vi "local FIFO 5 ch 8or12kHz resonance scanner (FPGA) fixed pix clock.vi"() -> ()   [LabVIEW 2012]
uses:
  <vilib>/eio/EIONode/EIONode.xnode
  <vilib>/rvi/eio/common/nirviEmuTemplateMethod_errors.vi
  <vilib>/rvi/DataTransferAndStorage/Container/XNode/niFpgaContainer.xnode
  <vilib>/platform/TimedLoop/XDataNode/XDataNode.xnode
  <vilib>/Platform/TimedLoop/XDataNode/nitl_modes.ctl
  <vilib>/Platform/TimedLoop/XDataNode/XDNodeRunTimeDep.lvlib
  <vilib>/Platform/TimedLoop/XDataNode/wakeup.ctl
  <vilib>/Platform/TimedLoop/XDataNode/timing_clust.ctl
  <vilib>/rvi/interface/RandomDataEmulation/nirviRandomDataFpgaReadWriteTemplate.vi
  <vilib>/rvi/FIFO/Fifo_Resource/nirvififoEmulationRead.vi
  <vilib>/rvi/FIFO/Fifo_Resource/nirvififoEmulationWrite.vi
panel:
  in  "frequency (T:8kHz F:12kHz)":bool
  in  "lines at once":i16=4999
  in  "Start Delay (Ticks)":i16 caption="Start delay (Ticks)"
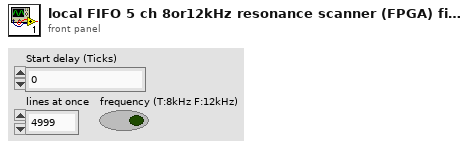
[diagram p1: front panel]
types:
  T1 = typedef "XDNodeRunTimeDep.lvlib/timing_clust.ctl" = cluster{"Expected End [f-1]":u64, "Actual End [f-1]":u64, "Finished Late? [f-1]":bool, "Expected End [i-1]":u64, "Actual End [i-1]":u64, "Finished Late? [i-1]":bool, "Expected Start [i]":u64, "Actual Start [i]":u64, "Expected Start [f]":u64, "Actual Start [f]":u64, "Source Name":string, "Structure Name":string, "Period":i64, "Deadline":i64, "Offset":i64, "Start":i64, "Priority":i32, "Timeout":i32, "Mode":T2, "Wakeup Reason":T3, "Error":errorcluster, "Source Type":string, "Secondary Source Type":string, "Global End Time":u64, "Global Start Time":u64, "Frame Duration":u64, "Iteration Duration":u64, "Assigned CPU":i32, "I/O Scan Engine Mode":u32}
  T2 = typedef "XDNodeRunTimeDep.lvlib/nitl_modes.ctl" = enum32{"No Change", "Process missed periods, maintain original phase", "Discard missed periods, maintain original phase", "Process missed periods, ignore original phase", "Discard missed periods, ignore original phase"}
  T3 = typedef "XDNodeRunTimeDep.lvlib/wakeup.ctl" = enum32{"Normal", "Aborted", "Asynchronous wakeup", "Timing source error", "Timed loop error", "Timeout"}
  T4 = cluster{"IO Module\\AI A0":i32, "IO Module\\AI A1":i32, "IO Module\\AI A3":i32, "IO Module\\AI A6":i32, "IO Module\\AI B8":i32}
  T5 = cluster{"IO Module\\AI A0":i16, "IO Module\\AI A1":i16, "IO Module\\AI A3":i16, "IO Module\\AI A6":i16, "IO Module\\AI B8":i16}
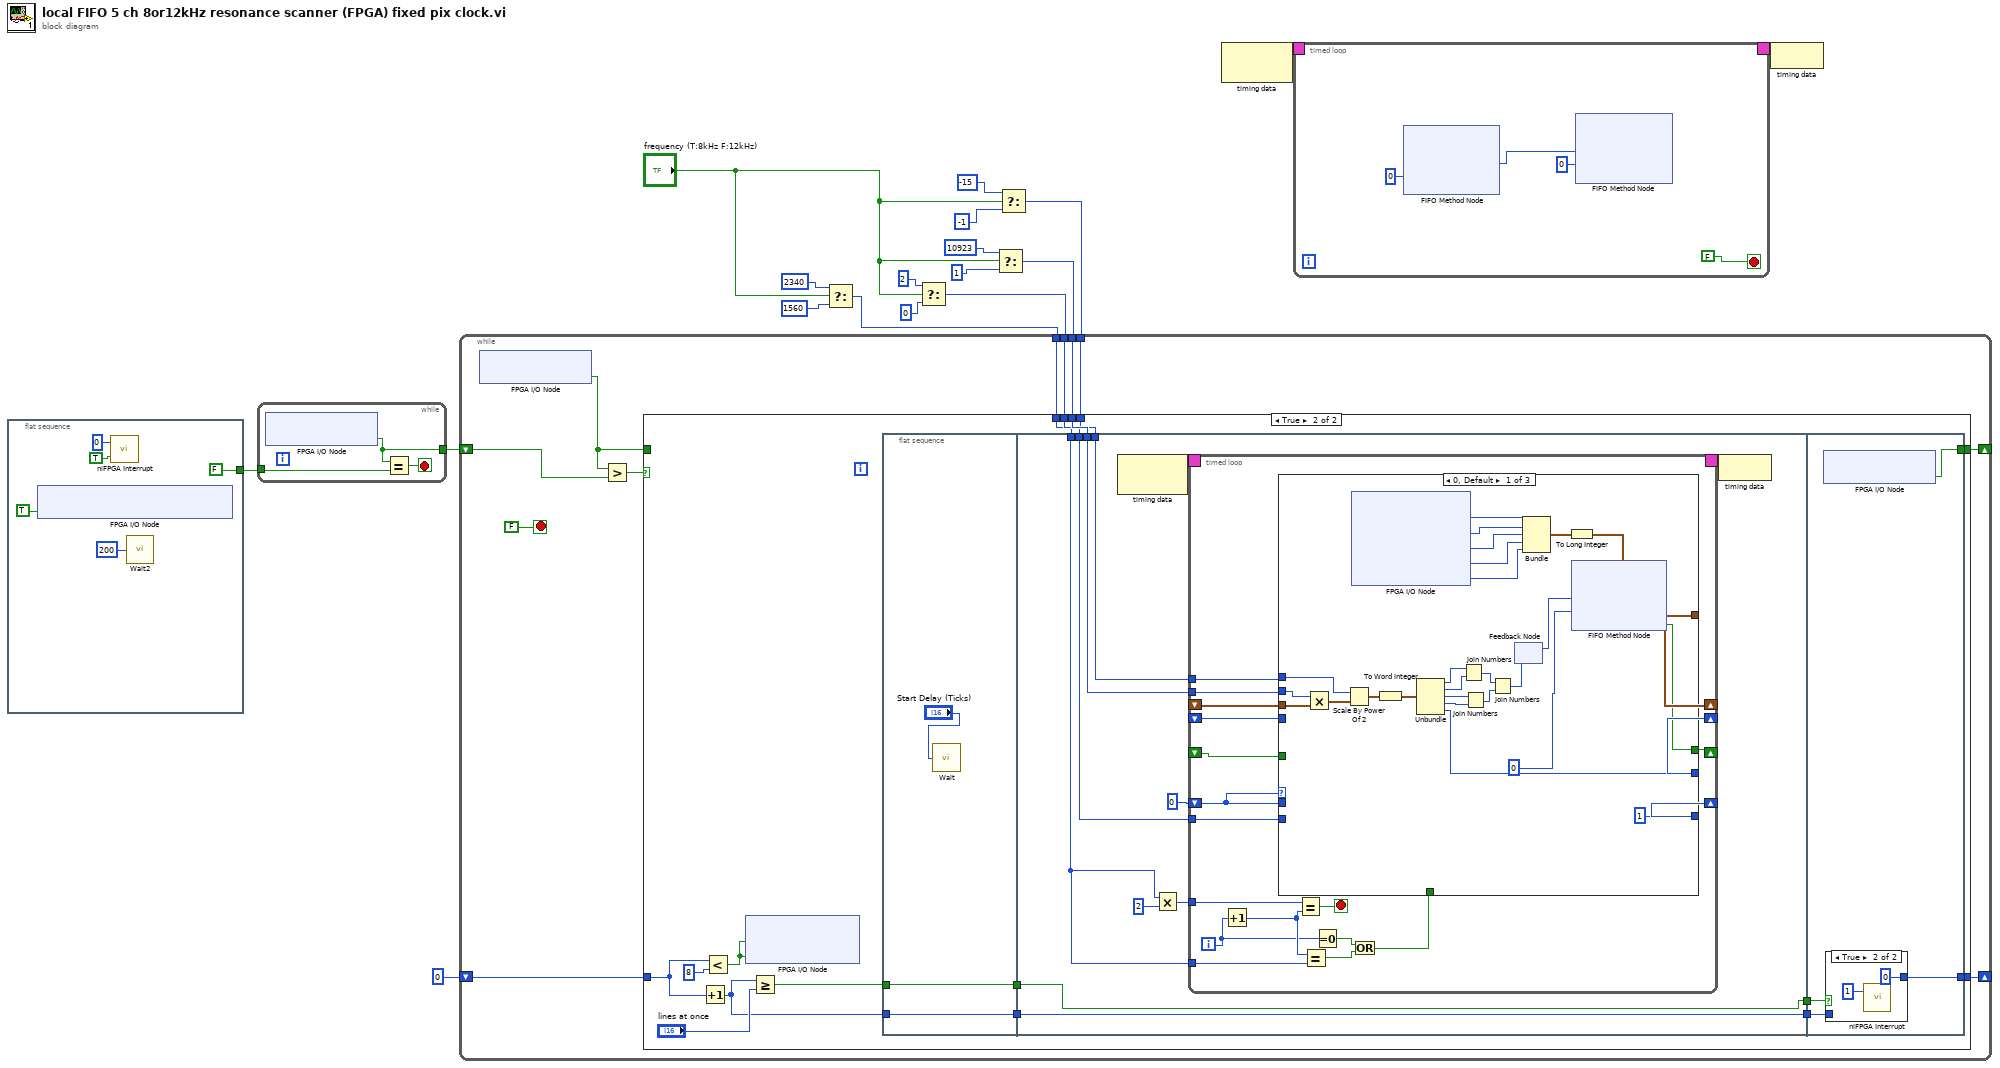
[diagram p0: block diagram]
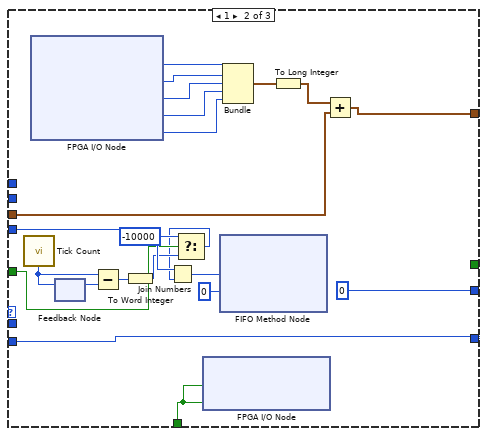
[diagram p3: hidden frame]
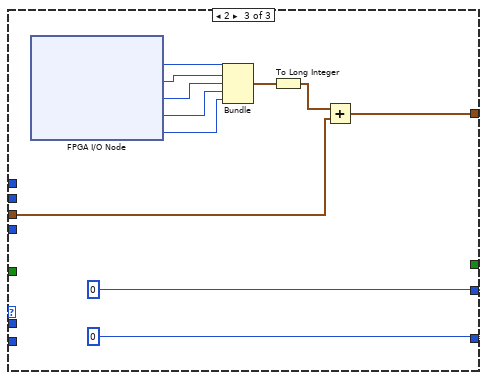
[diagram p4: hidden frame]
diagram:
  n1 = flat-sequence {
    tunnel: [FALSE ("IO Module\\DI 0")] -> w17
    frame #0 {
      n2 = xnode "FPGA I/O Node"("IO Module\\Digital Output Enable"=TRUE ("IO Module\\Digital Output Enable")) -> ()  [unwired: 1 in, 1 out]
      n3 = call <vilib>:"niFPGA Interrupt.vi"("Wait Until Cleared (F)"=TRUE, "IRQ Number (0)"=u8 0) -> ()  [unwired: 1 in]
      n4 = call "Wait2"("Count(mSec)"=u32 200) -> ()  [unwired: 1 out]
    }
  }
  n5 = while {
    tunnel: w17 -> [w26]
    tunnel: [w24] -> w16
    stop <- w25 stop-if-true
    n6 = xnode "FPGA I/O Node"() -> ("IO Module\\DI 0"=w24:bool)  [unwired: 1 in, 1 out]
    n7 = Equal?(x=w24, y=w26) -> (x = y?=w25:bool)
  }
  n8 = Select(t=i16 2340 ("samples per half period"), s="frequency (T:8kHz F:12kHz)", f=i16 1560 ("samples per half period")) -> (s? t:f=w3:i16)
  n9 = Select(t=i8 2 ("f"), s="frequency (T:8kHz F:12kHz)", f=i8 0 ("n")) -> (s? t:f=w7:i8)
  n10 = Select(t=i16 10923 ("n"), s="frequency (T:8kHz F:12kHz)", f=i16 1) -> (s? t:f=w9:i16)
  n11 = Select(t=i16 -15 ("n"), s="frequency (T:8kHz F:12kHz)", f=i16 -1 ("n")) -> (s? t:f=w8:i16)
  n12 = while {
    shift-right: [w36] -> _
    shift-left: w16 -> [w37]
    shift-right: [w34] -> _
    shift-left: i16 0 ("IRQ Number (0)") -> [w33]
    tunnel: w9 -> [w31]
    tunnel: w8 -> [w30]
    tunnel: w7 -> [w29]
    tunnel: w3 -> [w28]
    stop <- FALSE stop-if-true
    n13 = xnode "FPGA I/O Node"() -> ("IO Module\\DI 0"=w27:bool)  [unwired: 1 in, 1 out]
    n14 = Greater?(x=w27, y=w37) -> (0:w32:bool)
    n15 = case shown="True" w32 {
      tunnel: [w38 w52] -> w36
      tunnel: w33 -> [w39 w54]
      tunnel: [w39 w55] -> w34
      tunnel: w27 -> [w38 _]
      tunnel: w31 -> [_ w51]
      tunnel: w30 -> [_ w50]
      tunnel: w29 -> [_ w49]
      tunnel: w28 -> [_ w48]
      frame False {
      }
      frame True {
        n16 = Increment(x=w54) -> (x+1=w43:i16)
        n17 = Less?(x=w54, y=i16 8) -> (x < y?=w47:bool)
        n18 = xnode "FPGA I/O Node"("PXI_Trig2"=w47, "IO Module\\D0 2"=w47) -> ()  [unwired: 2 in, 2 out]
        n19 = Greater Or Equal?(x=w43, y="lines at once") -> (x >= y?=w40:bool)
        n20 = flat-sequence {
          tunnel: [w57] -> w44
          tunnel: w43 -> [w57]
          tunnel: [w56] -> w41
          tunnel: w40 -> [w56]
          tunnel: w51 -> [w64]
          tunnel: w50 -> [w63]
          tunnel: w49 -> [w62]
          tunnel: w48 -> [w61]
          tunnel: [w60] -> w45
          tunnel: w44 -> [w60]
          tunnel: [w59] -> w42
          tunnel: w41 -> [w59]
          tunnel: [w154] -> w55
          tunnel: [w153] -> w52
          tunnel: w45 -> [w152]
          tunnel: w42 -> [w151]
          frame #0 {
            n21 = call "Wait"("Count(Ticks)"="Start Delay (Ticks)") -> ()  [unwired: 1 out]
          }
          frame #1 {
            n22 = node-c288() -> (w67:T1)  [unwired: 1 in]
            n23 = Multiply(x=w61, y=i16 2) -> (x*y=w68:i16)
            n24 = timed-loop {
              tunnel: w68 -> [w87]
              timing: w67 -> [_]
              timing-out: [_] -> w66
              shift-right: [w86] -> _
              shift-left: i8 0 ("Timeout") -> [w76]
              tunnel: w61 -> [w82]
              shift-right: [w80] -> _
              shift-left: _ -> [w79]
              shift-right: [w78] -> _
              shift-left: _ -> [w77]
              tunnel: w64 -> [w75]
              tunnel: w63 -> [w74]
              tunnel: w62 -> [w73]
              shift-right: [w72] -> _
              shift-left: _ -> [w71]
              i -> [w81]
              stop <- w88 stop-if-true
              n25 = Increment(x=w81) -> (x+1=w83:i32)
              n26 = Equal?(x=w87, y=w83) -> (x = y?=w88:bool)
              n27 = Equal?(x=w83, y=w82) -> (x = y?=w84:bool)
              n28 = Equal To 0?(x=w81) -> (x = 0?=w85:bool)
              n29 = Or(x=w85, y=w84) -> (x .or. y?=w70:bool)
              n30 = case shown="0, Default" w76 {
                tunnel: w76 -> [_ _ _]
                tunnel: [i8 1 w115 i8 0] -> w86
                tunnel: [w107 w127 w138] -> w80
                tunnel: w79 -> [w98 w128 w139]
                tunnel: [w94 i16 0 ("IO Module\\AI B8") i16 0 ("IO Module\\AI B8")] -> w78
                tunnel: w77 -> [_ w122 _]
                tunnel: w75 -> [w97 _ _]
                tunnel: w74 -> [w96 _ _]
                tunnel: w73 -> [_ w115 _]
                tunnel: [w89 _ _] -> w72
                tunnel: w71 -> [_ w118 _]
                tunnel: w70 -> [_ w114 _]
                frame 0, Default {
                  n31 = Multiply(x=w97, y=w98) -> (x*y=w100:T4)
                  n32 = Scale By Power Of 2(n=w96, x=w100) -> (x*2^n=w99:T4)
                  n33 = xnode "FPGA I/O Node"() -> ("IO Module\\AI A0"=w113:i16, "IO Module\\AI A1"=w112:i16, "IO Module\\AI A3"=w111:i16, "IO Module\\AI A6"=w110:i16, "IO Module\\AI B8"=w108:i16)  [unwired: 5 in, 5 out]
                  n34 = To Word Integer(number=w99) -> (16bit integer=w95:T5)
                  n35 = Unbundle(w95) -> ("IO Module\\AI A0"=w104:i16, "IO Module\\AI A1"=w103:i16, "IO Module\\AI A3"=w102:i16, "IO Module\\AI A6"=w101:i16, "IO Module\\AI B8"=w94:i16)
                  n36 = Join Numbers(hi=w104, lo=w103) -> ((hi.lo)=w105:u32)
                  n37 = Join Numbers(hi=w102, lo=w101) -> ((hi.lo)=w106:u32)
                  n38 = Join Numbers(hi=w105, lo=w106) -> ((hi.lo)=w93:u64)
                  n39 = feedback-in #1(w93) -> ()
                  n40 = feedback #1() -> (w91:u64)  [unwired: 1 in]
                  n41 = Bundle("IO Module\\AI A0"=w113, "IO Module\\AI A1"=w112, "IO Module\\AI A3"=w111, "IO Module\\AI A6"=w110, "IO Module\\AI B8"=w108) -> (w109:T5)  [unwired: 1 in]
                  n42 = To Long Integer(number=w109) -> (32bit integer=w107:T4)
                  n43 = xnode ("FIFO Method Node")("Element"=w91, "Timeout"=0) -> ("Timed Out?"=w89:bool)  [unwired: 1 in, 1 out]
                }
                frame 1 {
                  n44 = call "Tick Count"() -> ("Tick Count(Ticks)"=w126:u32)
                  n45 = xnode "FPGA I/O Node"() -> ("IO Module\\AI A0"=w135:i16, "IO Module\\AI A1"=w134:i16, "IO Module\\AI A3"=w133:i16, "IO Module\\AI A6"=w132:i16, "IO Module\\AI B8"=w130:i16)  [unwired: 5 in, 5 out]
                  n46 = feedback #2() -> (w125:u32)  [unwired: 1 in]
                  n47 = feedback-in #2(w126) -> ()
                  n48 = Subtract(x=w126, y=w125) -> (x-y=w124:u32)
                  n49 = To Word Integer(number=w124) -> (16bit integer=w119:i16)
                  n50 = Select(t=i16 -10000, s=w118, f=w119) -> (s? t:f=w116:i16)
                  n51 = Join Numbers(hi=w122, lo=w116) -> ((hi.lo)=w120:u32)
                  n52 = xnode "FPGA I/O Node"("IO Module\\D0 1"=w114, "PXI_Trig1"=w114) -> ()  [unwired: 2 in, 2 out]
                  n53 = xnode ("FIFO Method Node")("Element"=w120, "Timeout"=0) -> ()  [unwired: 1 in, 2 out]
                  n54 = Bundle("IO Module\\AI A0"=w135, "IO Module\\AI A1"=w134, "IO Module\\AI A3"=w133, "IO Module\\AI A6"=w132, "IO Module\\AI B8"=w130) -> (w131:T5)  [unwired: 1 in]
                  n55 = To Long Integer(number=w131) -> (32bit integer=w129:T4)
                  n56 = Add(x=w129, y=w128) -> (x+y=w127:T4)
                }
                frame 2 {
                  n57 = xnode "FPGA I/O Node"() -> ("IO Module\\AI A0"=w146:i16, "IO Module\\AI A1"=w145:i16, "IO Module\\AI A3"=w144:i16, "IO Module\\AI A6"=w143:i16, "IO Module\\AI B8"=w141:i16)  [unwired: 5 in, 5 out]
                  n58 = Bundle("IO Module\\AI A0"=w146, "IO Module\\AI A1"=w145, "IO Module\\AI A3"=w144, "IO Module\\AI A6"=w143, "IO Module\\AI B8"=w141) -> (w142:T5)  [unwired: 1 in]
                  n59 = To Long Integer(number=w142) -> (32bit integer=w140:T4)
                  n60 = Add(x=w140, y=w139) -> (x+y=w138:T4)
                }
              }
            }
            n61 = node-c288(w66) -> ()
          }
          frame #2 {
            n62 = xnode "FPGA I/O Node"() -> ("IO Module\\DI 0"=w153:bool)  [unwired: 1 in, 1 out]
            n63 = case shown="True" w151 {
              tunnel: w152 -> [w155 _]
              tunnel: [w155 u8 0] -> w154
              frame False {
              }
              frame True {
                n64 = call <vilib>:"niFPGA Interrupt.vi"("IRQ Number (0)"=u8 1) -> ()  [unwired: 2 in]
              }
            }
          }
        }
      }
    }
  }
  n65 = node-c288() -> (w2:T1)  [unwired: 1 in]
  n66 = timed-loop {
    timing: w2 -> [_]
    timing-out: [_] -> w1
    stop <- FALSE stop-if-true
    n67 = xnode ("FIFO Method Node")("Timeout"=0) -> ("Element"=w160:u64)  [unwired: 1 in, 2 out]
    n68 = xnode ("FIFO Method Node")("Element"=w160, "Timeout"=0) -> ()  [unwired: 1 in, 2 out]
  }
  n69 = node-c288(w1) -> ()
